vi "mbug_2820_list.vi"() -> ()   [LabVIEW 2014]
uses:
  <instrlib>/MBUG-2820/MBUG-2820.lvlib
panel:
  out "Attached devices":i32[](listbox)
  # "MBUG-2820 list example"
  # "A list of available devices is assembled at VI start. Restart VI to refresh the list."
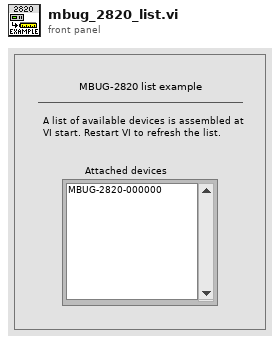
[diagram p1: front panel]
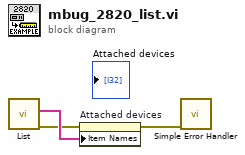
[diagram p0: block diagram]
diagram:
  n1 = call <instrlib>:"List.vi"() -> ("error out"=w2:errorcluster, "Device id strings"=w3:string[])  [unwired: 5 in, 1 out]
  n2 = property on="Attached devices" class="LstBox (strict)"(error in=w2, "Item Names"=w3) -> (error out=w1:errorcluster)  [unwired: 1 in, 1 out]
  n3 = call <vilib>:"Simple Error Handler.vi"("error in (no error)"=w1) -> ()  [unwired: 4 in, 5 out]
